vi "To ServoPWM.vi"(2 "error in (no error)":errorcluster, 3 "Wheel Angle":dbl, 4 "Car.lvclass 2":refnum<class "Car.lvclass">) -> (0 "error out":errorcluster, 1 "ServoPWM":dbl)   [LabVIEW 2015, in "Car.lvclass"]
uses:
  Car.lvclass
  Car.lvclass/Car.ctl
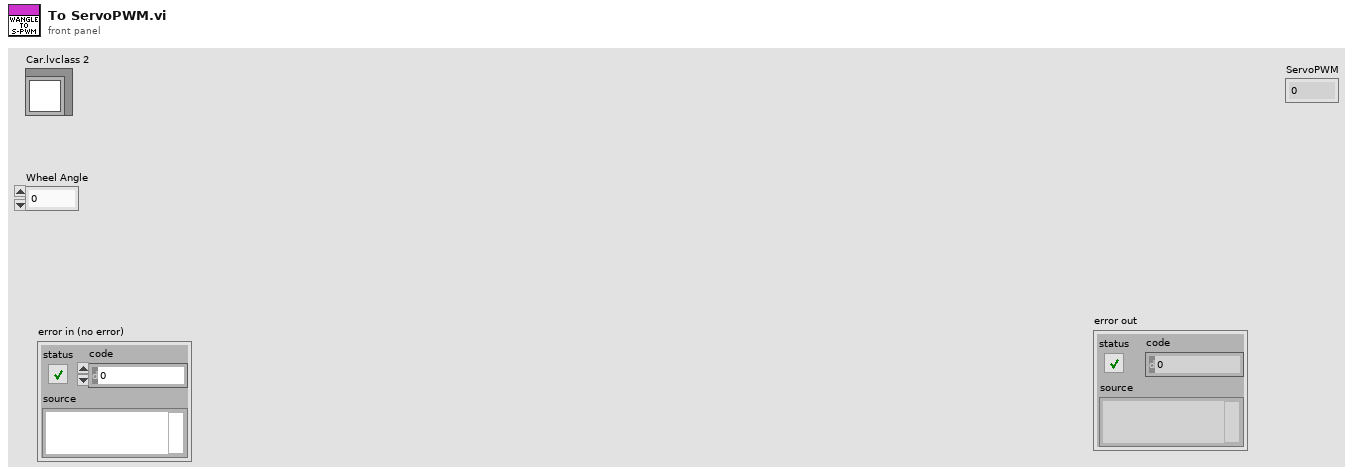
[diagram p1: front panel]
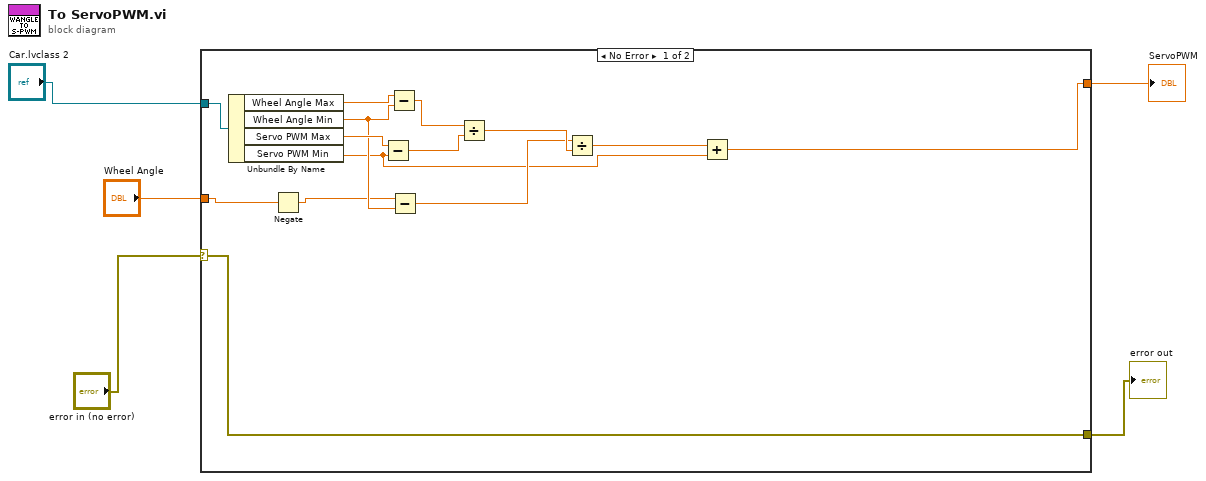
[diagram p0: block diagram]
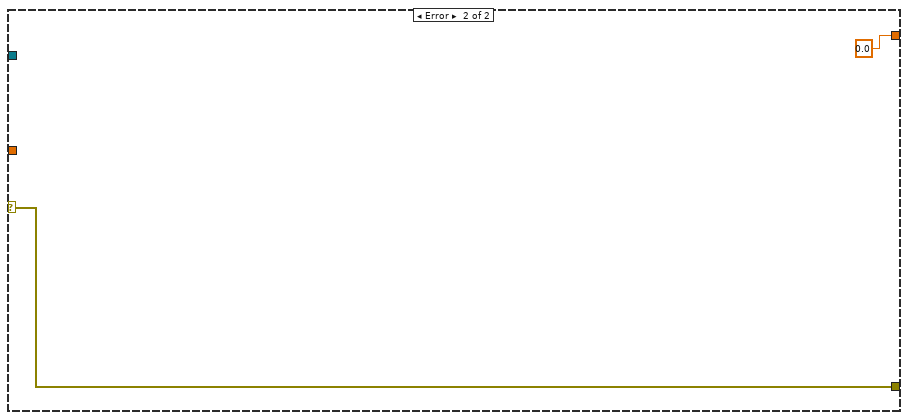
[diagram p2: hidden frame]
diagram:
  n1 = case shown="No Error" "error in (no error)" {
    selector: "error in (no error)" -> [w19 w21]
    tunnel: [w19 w21] -> w4
    tunnel: [w8 0.0] -> w3
    tunnel: "Car.lvclass 2" -> [w18 _]
    tunnel: "Wheel Angle" -> [w7 _]
    frame No Error {
      n2 = Unbundle By Name(w18) -> ("Wheel Angle Max"=w17:dbl, "Wheel Angle Min"=w12:dbl, "Servo PWM Max"=w16:dbl, "Servo PWM Min"=w9:dbl)
      n3 = Negate(x=w7) -> (-x=w6:dbl)
      n4 = Subtract(x=w16, y=w9) -> (x-y=w14:dbl)
      n5 = Subtract(x=w17, y=w12) -> (x-y=w15:dbl)
      n6 = Subtract(x=w6, y=w12) -> (x-y=w11:dbl)
      n7 = Divide(x=w15, y=w14) -> (x/y=w13:dbl)
      n8 = Divide(x=w11, y=w13) -> (x/y=w10:dbl)
      n9 = Add(x=w10, y=w9) -> (x+y=w8:dbl)
    }
    frame Error {
    }
  }
  "ServoPWM" <- w3
  "error out" <- w4
